vi "Halt.vi"(8 "error in (no error)":errorcluster, 11 "UDP Reader in":refnum<class "UDP Reader.lvclass">) -> (0 "error out":errorcluster, 3 "UDP Reader out":refnum<class "UDP Reader.lvclass">)   [LabVIEW 2022 SP3, in "UDP Reader.lvlib" / "UDP Reader.lvclass"]
uses:
  UDP Reader.lvclass
  UDP Reader.lvclass/UDP Reader.ctl
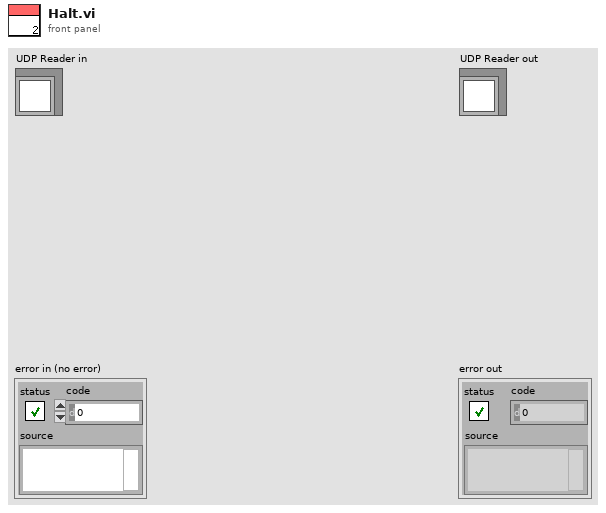
[diagram p1: front panel]
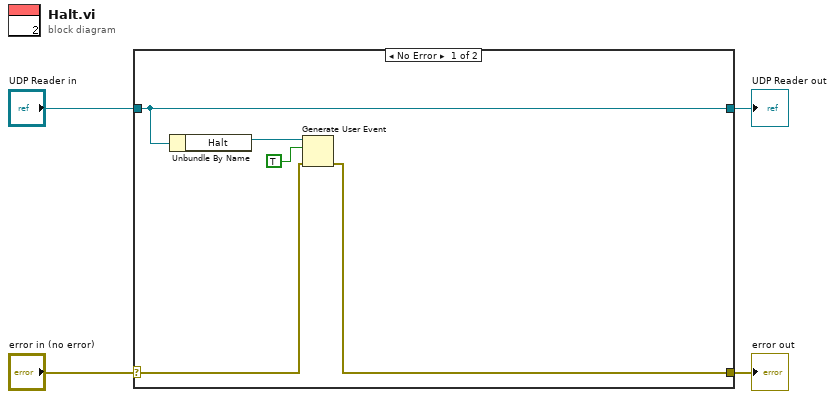
[diagram p0: block diagram]
diagram:
  n1 = case shown="No Error" "error in (no error)" {
    selector: "error in (no error)" -> [w6 w11]
    tunnel: [w7 w11] -> w3
    tunnel: [w9 w10] -> w1
    tunnel: "UDP Reader in" -> [w9 w10]
    frame No Error {
      n2 = Unbundle By Name(w9) -> ("Halt"=w8:refnum<user-event>)
      n3 = Generate User Event(user event=w8, event data cluster=TRUE ("event data"), error in=w6) -> (error out=w7:errorcluster)  [unwired: 1 in, 1 out]
    }
    frame Error {
    }
  }
  "error out" <- w3
  "UDP Reader out" <- w1
